vi "x-values.vi"(1 "TAC Gain":i16, 2 "TAC Rang [ns]":sgl format="%.2f", 3 "No. Microchannel":i32) -> (0 "Array":dbl[](array[numeric]) format="%.2f")   [LabVIEW 2009]
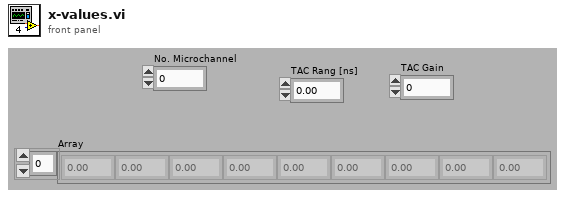
[diagram p1: front panel]
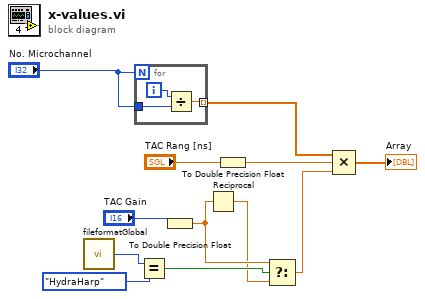
[diagram p0: block diagram]
diagram:
  n1 = call "fileformatGlobal.vi"() -> ("fileformat out"=w6:enum16{"Herty", "Ken", "SPC130", "HydraHarp"})  [unwired: 2 in]
  n2 = for {
    N: "No. Microchannel" -> [_]
    tunnel: [w13] -> w8 mode=indexing
    tunnel: "No. Microchannel" -> [w15]
    i -> [w14]
    n3 = Divide(x=w14, y=w15) -> (x/y=w13:dbl)
  }
  n4 = Equal?(x=w6, y=enum16{"Herty", "Ken", "SPC130", "HydraHarp"}."HydraHarp") -> (x = y?=w4:bool)
  n5 = To Double Precision Float(number="TAC Gain") -> (double precision float=w3:dbl)
  n6 = Reciprocal(x=w3) -> (1/x=w2:dbl)
  n7 = To Double Precision Float(number="TAC Rang [ns]") -> (double precision float=w7:dbl)
  n8 = Select(t=w3, s=w4, f=w2) -> (s? t:f=w1:dbl)
  n9 = Compound Arithmetic op=MULTIPLY(w8, w7, w1) -> (→"Array":dbl[])
